vi "Test.vi"() -> ()   [LabVIEW 2018]
panel:
  out "error out":errorcluster
  out "Q":i16[](array[numeric])
  out "I":i16[](array[numeric])
  in  "Param":T1
  in  "RFIndex":u32
  in  "Path":path
  in  "error in (no error)":errorcluster
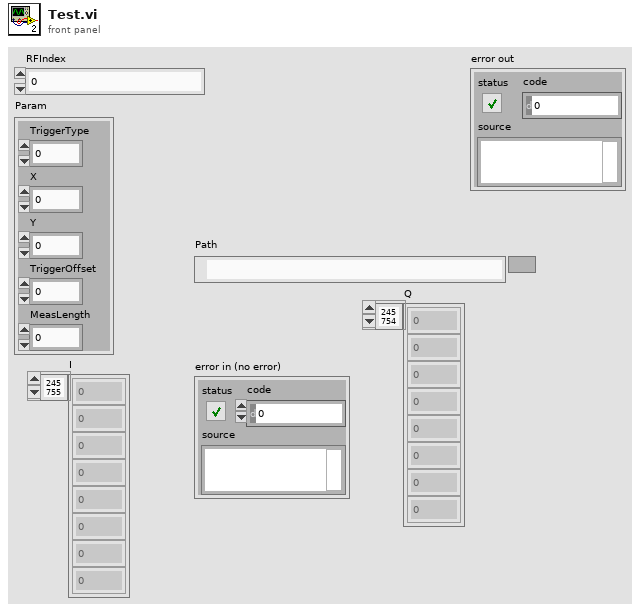
[diagram p1: front panel]
types:
  T1 = cluster{"TriggerType":dbl, "X":dbl, "Y":dbl, "TriggerOffset":dbl, "MeasLength":dbl}
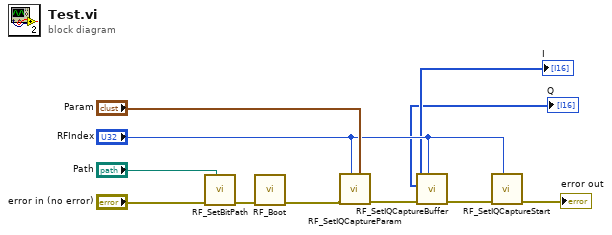
[diagram p0: block diagram]
diagram:
  n1 = call "RF_SetBitPath.vi"("Path"="Path", "error in (no error)"="error in (no error)") -> ("error out"=w9:errorcluster)  [unwired: 8 in, 1 out]
  n2 = call "RF_Boot.vi"("error in (no error)"=w9) -> ("error out"=w8:errorcluster)  [unwired: 9 in, 1 out]
  n3 = call "RF_SetIQCaptureParam.vi"("Param"="Param", "RFIndex"="RFIndex", "Error In"=w8) -> ("Error Out"=w6:errorcluster)  [unwired: 7 in, 1 out]
  n4 = call "RF_SetIQCaptureBuffer.vi"("RFIndex"="RFIndex", "error in (no error)"=w6) -> ("error out"=w5:errorcluster, "Q"=→"Q":i16[], "I"=→"I":i16[])  [unwired: 6 in, 1 out]
  n5 = call "RF_SetIQCaptureStart.vi"("RFIndex"="RFIndex", "error in (no error)"=w5) -> ("error out"=→"error out":errorcluster)  [unwired: 8 in, 1 out]
